vi "Timeout.vi"(8 "error in (no error)":errorcluster, 11 "Cylinder in":refnum<class "Cylinder.lvclass">) -> (0 "error out":errorcluster, 3 "Cylinder out":refnum<class "Cylinder.lvclass">)   [LabVIEW 2015, in "cRIO-Carbondioxide.lvlib" / "CO2-Actor.lvlib" / "Cylinder.lvclass"]
uses:
  Cylinder.lvclass
  CO2 Actor/CO2 Actor.lvclass
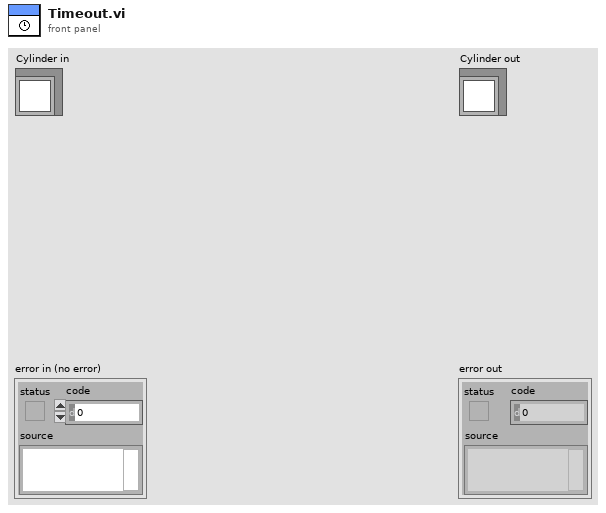
[diagram p1: front panel]
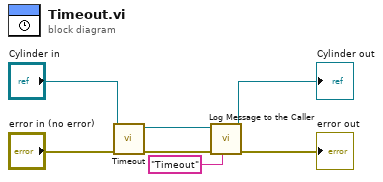
[diagram p0: block diagram]
diagram:
  n1 = call-parent "Timeout.vi"("error in (no error)"="error in (no error)", "CO2 Actor in"="Cylinder in") -> ("error out"=w5:errorcluster, "CO2 Actor out"=w3:refnum<class "Cylinder.lvclass">)  [unwired: 8 in]
  n2 = call-dynamic "Log Message to the Caller.vi"("String (\"\" = no message to send)"="Timeout" ("String (\"\" = no message to send)"), "error in (no error)"=w5, "CO2 Actor in"=w3) -> ("error out"=→"error out":errorcluster, "CO2 Actor out"=→"Cylinder out":refnum<class "Cylinder.lvclass">)  [unwired: 7 in]
